vi "Periodic Tasks.vi"(8 "error in":errorcluster) -> ()   [LabVIEW 2012]
doc: "This VI runs in parallel to other tasks. It can contain as many user-defined periodic loops as you need. These can carry out PID or other sorts of timed response."
uses:
  <vilib>/Rock Robotics/SystemInterfaces/Utilities/FPGA_UtilitiesLED Source.ctl
  <vilib>/Rock Robotics/SystemInterfaces/Utilities/FPGA_UtilitiesLED State.ctl
  <vilib>/Rock Robotics/WPI/DriverStation/WPI_DriverStationRobotMode2.ctl
  Robot Global Data.vi
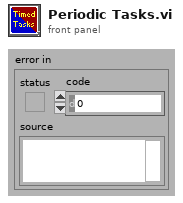
[diagram p1: front panel]
types:
  T1 = typedef "WPI_DriverStationRobotMode2.ctl" = enum16{"Autonomous Disabled", "Autonomous Enabled", "Teleop Disabled", "Teleop Enabled", "Timeout", "Finish", "Test Disabled", "Test Enabled"}
  T2 = cluster{"Joy Stick":cluster{"Secondary":cluster{"Buttons":cluster{"A":bool, "B":bool, "X":bool, "Y":bool, "Left Bumper":bool, "Right Bumper":bool, "Back":bool, "Start":bool, "Left Thumbstick":bool, "Right Thumbstick":bool}, "Axes":cluster{"Left Stick X ":dbl, "Left Stick Y":dbl, "Triggers":dbl, "Right Stick X":dbl, "Right Stick Y":dbl, "D-Pad X":dbl}}, "Primary":cluster{"Buttons":cluster{"A":bool, "B":bool, "X":bool, "Y":bool, "Left Bumper":bool, "Right Bumper":bool, "Back":bool, "Start":bool, "Left Thumbstick":bool, "Right Thumbstick":bool}, "Axes":cluster{"Left Stick X ":dbl, "Left Stick Y":dbl, "Triggers":dbl, "Right Stick X":dbl, "Right Stick Y":dbl, "D-Pad X":dbl}}}, "Arm":cluster{"Arm Set":dbl, "Arm Current":dbl, "At Position?":bool}, "Drive":cluster{"Right":dbl, "Left":dbl}, "Shooter":cluster{"RPM Current":dbl, "RPM Set":dbl, "In Range?":bool}, "Climb State":enum16{"Arm Up", "Arm Down", "Arm Attach", "Arm Wait"}, "EncodeReset":bool}
  T3 = enum16{"Arm Up", "Arm Down", "Arm Attach", "Arm Wait"}
  T4 = typedef "FPGA_UtilitiesLED State.ctl" = enum16{"Off", "On", "Toggle"}
  T5 = typedef "FPGA_UtilitiesLED Source.ctl" = enum16{"User LED", "FPGA LED"}
  T6 = typedef "WPI_CompressorDevRef.ctl" = cluster{"DevStatus":errorcluster, "DigitalInputDevRef":T7, "RelayDevRef":T10}
  T7 = typedef "WPI_DigitalInputDevRef.ctl" = cluster{"DevStatus":errorcluster, "DIO Channel":T8, "Digital Module":T9}
  T8 = typedef "FPGA_DIOChannel.ctl" = enum8{"DIO 1", "DIO 2", "DIO 3", "DIO 4", "DIO 5", "DIO 6", "DIO 7", "DIO 8", "DIO 9", "DIO 10", "DIO 11", "DIO 12", "DIO 13", "DIO 14", "Invalid"}
  T9 = typedef "FPGA_TypedefDigitalModule.ctl" = enum16{"Digital Module 1", "Digital Module 2"}
  T10 = typedef "WPI_RelayDevRef.ctl" = cluster{"DevStatus":errorcluster, "Relay Channel":T11, "Digital Module":T9, "Relay Direction":T12}
  T11 = typedef "FPGA_DIORelayChannel.ctl" = enum8{"Relay 1", "Relay 2", "Relay 3", "Relay 4", "Relay 5", "Relay 6", "Relay 7", "Relay 8", "Invalid"}
  T12 = typedef "WPI_RelayDirection.ctl" = enum16{"Both directions", "Forward only", "Reverse only"}
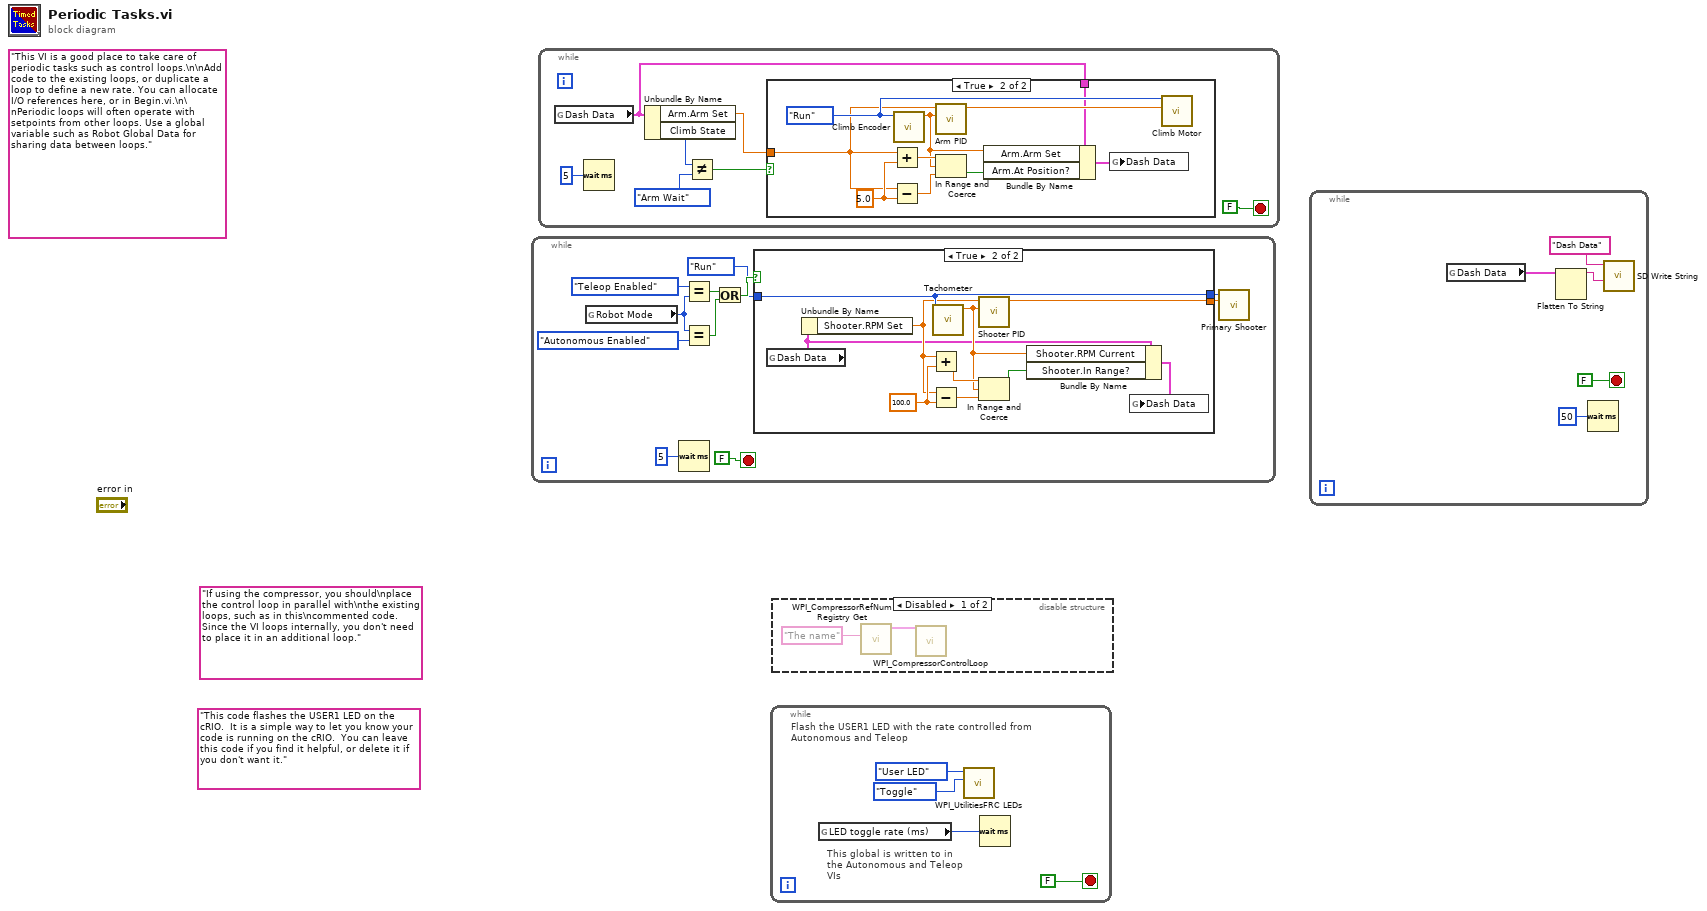
[diagram p0: block diagram]
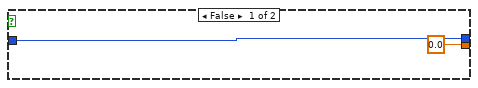
[diagram p3: hidden frame]
diagram:
  (unwired) "If using the compressor, you should\nplace the control loop in parallel with\nthe existing loops, such as in this\ncommented code. Since the VI loops internally, you don't need to place it in an additional loop."
  (unwired) "This code flashes the USER1 LED on the cRIO.  It is a simple way to let you know your code is running on the cRIO.  You can leave this code if you find it helpful, or delete it if you don't want it."
  (unwired) "This VI is a good place to take care of periodic tasks such as control loops.\n\nAdd code to the existing loops, or duplicate a loop to define a new rate. You can allocate I/O references here, or in Begin.vi.\n\nPeriodic loops will often operate with setpoints from other loops. Use a global variable such as Robot Global Data for sharing data between loops."
  n1 = while {
    stop <- FALSE stop-if-true
    n2 = global read "Robot Global Data.vi" "Robot Mode"() -> (w8:T1)
    n3 = Wait (ms)(milliseconds to wait=u32 5) -> ()  [unwired: 1 out]
    n4 = Equal?(x=WPI_DriverStationRobotMode2."Teleop Enabled" ("Robot Mode"), y=w8) -> (x = y?=w7:bool)
    n5 = Equal?(x=w8, y=WPI_DriverStationRobotMode2."Autonomous Enabled" ("Robot Mode")) -> (x = y?=w6:bool)
    n6 = Or(x=w7, y=w6) -> (x .or. y?=w4:bool)
    n7 = case shown="True" w4 {
      tunnel: enum16{"Start", "Run", "End"}."Run" ("Enum") -> [w12 w22]
      tunnel: [0.0 ("Shooter Motor") w23] -> w2
      tunnel: [w12 w22] -> w1
      frame False {
      }
      frame True {
        w20 = 100.0 ("y")
        n8 = global read "Robot Global Data.vi" "Dash Data"() -> (w14:T2)
        n9 = Unbundle By Name(w14) -> ("Shooter.RPM Set"=w17:dbl)
        n10 = Add(x=w17, y=w20) -> (x+y=w21:dbl)
        n11 = Subtract(x=w17, y=w20) -> (x-y=w19:dbl)
        n12 = call "Tachometer.vi"("Enum"=w22) -> ("RPM Current"=w16:dbl)  [unwired: 10 in]
        n13 = call "Shooter PID.vi"("RPM Current"=w16, "RPM Set"=w17) -> ("Shooter Motor"=w23:dbl)  [unwired: 9 in]
        n14 = In Range and Coerce(upper limit=w21, x=w16, lower limit=w19) -> (In Range?=w15:bool)  [unwired: 1 out]
        n15 = Bundle By Name(cluster=w14, "Shooter.RPM Current"=w16, "Shooter.In Range?"=w15) -> (w18:T2)
        n16 = global write "Robot Global Data.vi" "Dash Data"(w18) -> ()
      }
    }
    n17 = call "Primary Shooter.vi"("Motor Speed"=w2, "Enum"=w1) -> ()  [unwired: 10 in]
  }
  n18 = while {
    stop <- FALSE stop-if-true
    n19 = global read "Robot Global Data.vi" "Dash Data"() -> (w24:T2)
    n20 = Wait (ms)(milliseconds to wait=u32 5) -> ()  [unwired: 1 out]
    n21 = Unbundle By Name(w24) -> ("Arm.Arm Set"=w28:dbl, "Climb State"=w27:T3)
    n22 = Not Equal?(x=w27, y=T3."Arm Wait") -> (x != y?=w25:bool)
    n23 = case shown="True" w25 {
      tunnel: w28 -> [_ w32]
      tunnel: w24 -> [_ w31]
      frame False {
      }
      frame True {
        w37 = 5.0 ("y")
        w40 = enum16{"Start", "Run", "End"}."Run" ("Enum")
        n24 = Add(x=w32, y=w37) -> (x+y=w38:dbl)
        n25 = Subtract(x=w32, y=w37) -> (x-y=w36:dbl)
        n26 = call "Climb Encoder.vi"("Enum"=w40) -> ("Distance"=w33:dbl)  [unwired: 10 in]
        n27 = call "Arm PID.vi"("Arm Current"=w33, "Arm Set"=w32) -> ("Shooter Motor"=w39:dbl)  [unwired: 9 in]
        n28 = In Range and Coerce(upper limit=w38, x=w33, lower limit=w36) -> (In Range?=w34:bool)  [unwired: 1 out]
        n29 = Bundle By Name(cluster=w31, "Arm.Arm Set"=w33, "Arm.At Position?"=w34) -> (w35:T2)
        n30 = global write "Robot Global Data.vi" "Dash Data"(w35) -> ()
        n31 = call "Climb Motor.vi"("Output"=w39, "Enum"=w40) -> ()  [unwired: 10 in]
      }
    }
  }
  n32 = while {
    stop <- FALSE stop-if-true
    # "This global is written to in the Autonomous and Teleop VIs"
    # "Flash the USER1 LED with the rate controlled from Autonomous and Teleop"
    n33 = global read "Robot Global Data.vi" "LED toggle rate (ms)"() -> (w41:u32)
    n34 = call <vilib>:"WPI_UtilitiesFRC LEDs.vi"("State"=FPGA_UtilitiesLED_State."Toggle", "LED Type"=FPGA_UtilitiesLED_Source."User LED") -> ()  [unwired: 1 in, 9 out]
    n35 = Wait (ms)(milliseconds to wait=w41) -> ()  [unwired: 1 out]
  }
  n36 = disable-structure shown="Disabled" {
    frame Disabled {
      n37 = call <vilib>:"WPI_CompressorRefNum Registry Get.vi"("refnum name"="The name") -> ("CompressorDevRef"=w46:T6)  [unwired: 9 in, 1 out]
      n38 = call <vilib>:"WPI_CompressorControlLoop.vi"("CompressorDevRef"=w46) -> ()  [unwired: 11 in]
    }
    frame Enabled {
    }
  }
  n39 = while {
    stop <- FALSE stop-if-true
    n40 = global read "Robot Global Data.vi" "Dash Data"() -> (w47:T2)
    n41 = Flatten To String(anything=w47) -> (data string=w48:string)  [unwired: 3 in, 2 out]
    n42 = Wait (ms)(milliseconds to wait=u32 50) -> ()  [unwired: 1 out]
    n43 = call <vilib>:"SD Write String.vi"("String"=w48, "Name"="Dash Data") -> ()  [unwired: 8 in, 2 out]
  }
